vi "SubVI_Identificador_QRCode.vi"(8 "error in":errorcluster, 10 "ROI Objeto":T4 {"Contours"."Type" items=["No Selection", "Point", "Line", "Rectangle", "Oval", "Polygon", "Freehand Region", "Annulus", "Unused2", "Unused3", "Broken Line", "Freehand Line", "Rotated Rectangle"]}, 11 "Session In":T9) -> (0 "error out":errorcluster, 3 "Data":string)   [LabVIEW 2017]
uses:
  <vilib>/userdefined/High Color/IMAQdx.ctl
  <vilib>/vision/Instrument.llb/QR Code Search Options.ctl
  <vilib>/vision/Instrument.llb/Demodulation Mode.ctl
  <vilib>/vision/Instrument.llb/Cell Sample Size.ctl
  <vilib>/vision/Instrument.llb/Cell Filter Mode.ctl
  <vilib>/vision/Instrument.llb/QR Code Description Options.ctl
  <vilib>/vision/Instrument.llb/Data Matrix Polarity.ctl
  <vilib>/vision/Instrument.llb/QR Code Model Type.ctl
  <vilib>/vision/driver/IMAQdx.llb/IMAQdx Buffer Number Mode.ctl
  <vilib>/vision/driver/NI_Vision_Acquisition_Software.lvlib
  <vilib>/vision/NI_Vision_Development_Module.lvlib
panel:
  in  "QR Description Options":T1={"Matrix Size (cells)"=0, "Barcode Polarity"=-2, "Mirror Mode"=0, "QR Model"=3} {"Mirror Mode" items=["Auto-detect"=-2, "Normal"=0, "Mirrored"=1]; "Matrix Size (cells)" items=["Auto-detect"=0, "11x11 - Version 1 (Micro QR Only)"=11, "13x13 - Version 2 (Micro QR Only)"=13, "15x15 - Version 3 (Micro QR Only)"=15, "17x17 - Version 4 (Micro QR Only)"=17, "21x21 - Version 1"=21, "25x25 - Version 2"=25, "29x29 - Version 3"=29, "33x33 - Version 4"=33, "37x37 - Version 5"=37, "41x41 - Version 6"=41, "45x45 - Version 7"=45, "49x49 - Version 8"=49, "53x53 - Version 9"=53, "57x57 - Version 10"=57, "61x61 - Version 11"=61, "65x65 - Version 12"=65, "69x69 - Version 13"=69, "73x73 - Version 14"=73, "77x77 - Version 15"=77, "81x81 - Version 16"=81, "85x85 - Version 17"=85, "89x89 - Version 18"=89, "93x93 - Version 19"=93, "97x97 - Version 20"=97, "101x101 - Version 21"=101, "105x105 - Version 22"=105, "109x109 - Version 23"=109, "113x113 - Version 24"=113, "117x117 - Version 25"=117, "121x121 - Version 26"=121, "125x125 - Version 27"=125, "129x129 - Version 28"=129, "133x133 - Version 29"=133, "137x137 - Version 30"=137, "141x141 - Version 31"=141, "145x145 - Version 32"=145, "149x149 - Version 33"=149, "153x153 - Version 34"=153, "157x157 - Version 35"=157, "161x161 - Version 36"=161, "165x165 - Version 37"=165, "169x169 -  Version 38"=169, "173x173 - Version 39"=173, "177x177 - Version 40"=177]; "QR Model" items=["Auto-detect", "Micro", "Model 1", "Model 2"]; "Barcode Polarity" items=["Auto-detect"=-2, "Black on White"=0, "White on Black"=1]}
  in  "QR Search Options":T5={"Rotation Mode"=enum."Unlimited", "Skip Location?"=FALSE, "Edge Threshold"=30, "Demodulation Mode"=0, "Cell Sample Size"=-2, "Cell Filter Mode"=0, "Skew Degrees Allowed"=5} {"Cell Filter Mode" items=["Auto-detect"=-2, "Average"=0, "Median"=1, "Central Average"=2, "High Average"=3, "Low Average"=4, "Very High Average"=5, "Very Low Average"=6, "All Filters"=8]; "Cell Sample Size" items=["Auto-detect"=-2, "1x1"=1, "2x2"=2, "3x3"=3, "4x4"=4, "5x5"=5, "6x6"=6, "7x7"=7]; "Demodulation Mode" items=["Auto-detect"=-2, "Histogram"=0, "Local Contrast"=1, "Combination"=2, "All"=3]}
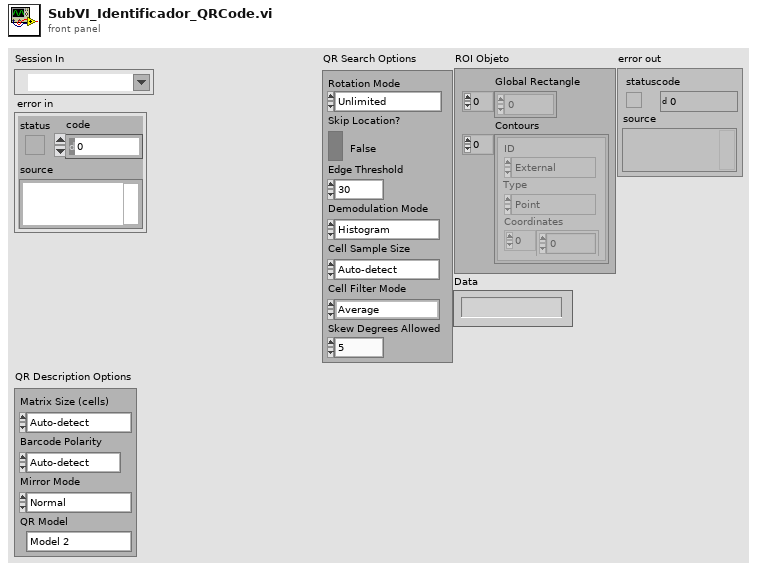
[diagram p1: front panel]
types:
  T1 = typedef "QR Code Description Options.ctl" = cluster{"Matrix Size (cells)":i32, "Barcode Polarity":T2, "Mirror Mode":i32, "QR Model":T3}
  T2 = typedef "Data Matrix Polarity.ctl" = i32
  T3 = typedef "QR Code Model Type.ctl" = i32
  T4 = typedef "ROI Descriptor" = cluster{"Global Rectangle":i32[], "Contours":cluster{"ID":enum32{"External", "Internal"}, "Type":u32, "Coordinates":i32[]}[]}
  T5 = typedef "QR Code Search Options.ctl" = cluster{"Rotation Mode":enum32{"Unlimited", "0 Degrees", "90 Degrees", "180 Degrees", "270 Degrees"}, "Skip Location?":bool, "Edge Threshold":u32, "Demodulation Mode":T6, "Cell Sample Size":T7, "Cell Filter Mode":T8, "Skew Degrees Allowed":u32}
  T6 = typedef "Demodulation Mode.ctl" = i32
  T7 = typedef "Cell Sample Size.ctl" = i32
  T8 = typedef "Cell Filter Mode.ctl" = i32
  T9 = typedef "IMAQdx.ctl" = refnum<k21>
  T10 = typedef "NI_Vision_Acquisition_Software.lvlib/IMAQdx Buffer Number Mode.ctl" = enum32{"Next", "Last", "Buffer Number", "Every", "Last New"}
  T11 = typedef "IMAQ Image.ctl" = refnum<image>
  T12 = typedef "QR Code Report.ctl" = cluster{"Found?":bool, "Data":string, "Bounding Box":cluster{"x":sgl, "y":sgl}[], "Errors Corrected":u32, "Dimensions (Rows/Cols)":u32, "Version":u32, "QR Model":T3, "Stream Mode":T13, "Barcode Polarity":T2, "Mirrored?":bool, "Append Stream Position":u32, "Size of Append Stream":u32, "First EAN-128 ID":i32, "First Alternate Language ID":i32, "Append Stream ID":u32, "Minimum Edge Strength":u32, "Demodulation Mode":T6, "Cell Sample Size":T7, "Cell Filter Mode":T8}
  T13 = typedef "QR Code Stream Mode Type.ctl" = i32
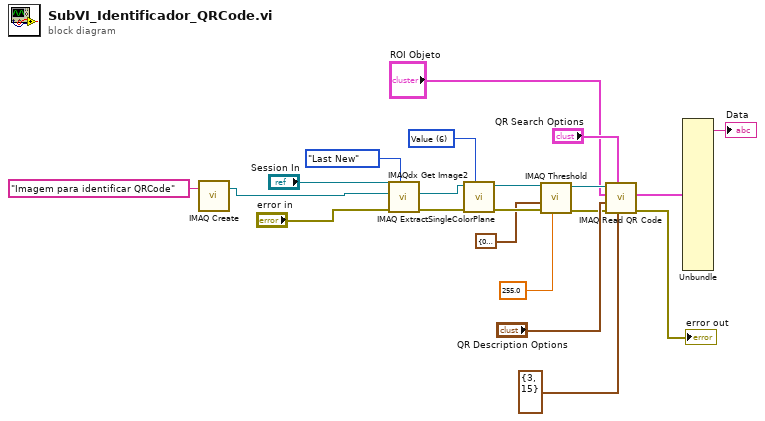
[diagram p0: block diagram]
diagram:
  w15 = 6 items=["Red", "Green", "Blue", "Hue", "Saturation", "Luminance", "Value", "Intensity"] ("Color Plane")
  n1 = call "IMAQ Create"("Image Name"="Imagem para identificar QRCode") -> ("New Image"=w17:T11)  [unwired: 4 in, 1 out]
  n2 = call <vilib>:"IMAQdx Get Image2.vi"("Buffer Number Mode (Next)"=IMAQdx_Buffer_Number_Mode."Last New", "error in"="error in", "Image In"=w17, "Session In"="Session In") -> ("error out"=w6:errorcluster, "Image Out"=w16:T11)  [unwired: 4 in, 2 out]
  n3 = call "IMAQ ExtractSingleColorPlane"("Color Plane"=w15, "error in (no error)"=w6, "Image Src"=w16) -> ("error out"=w5:errorcluster, "Image Dst Out"=w13:T11)  [unwired: 1 in, 6 out]
  n4 = call "IMAQ Threshold"("Replace Value"=sgl 255.0, "error in (no error)"=w5, "Range"=cluster{"Lower value":sgl, "Upper value":sgl} {"Lower value"=0.0, "Upper value"=150.0}, "Image Src"=w13) -> ("error out"=w4:errorcluster, "Image Dst Out"=w11:T11)  [unwired: 2 in, 4 out]
  n5 = call "IMAQ Read QR Code"("QR Code Cell Size (pixels)"=cluster{"Minimum Size":u32, "Maximum Size":u32} {"Minimum Size"=3, "Maximum Size"=15}, "QR Search Options"="QR Search Options", "error in (no error)"=w4, "QR Description Options"="QR Description Options", "ROI Descriptor"="ROI Objeto", "Image"=w11) -> ("error out"=→"error out":errorcluster, "QR Code Report"=w7:T12)  [unwired: 1 in, 3 out]
  n6 = Unbundle(w7) -> ("Data"=→"Data":string)  [unwired: 18 out]
